vi "CSM - Data Type.vi"(8 "error in (no error)":errorcluster, 11 "variant":variant) -> (0 "error out":errorcluster, 3 "Data Type String":string)   [LabVIEW 2017, in "CSM MassData Parameter Support.lvlib"]
uses:
  CSM MassData Parameter Support.lvlib
  <vilib>/Utility/Data Type/Type Definitions/Data Type.ctl
  <vilib>/Utility/Data Type/NI_Data Type.lvlib
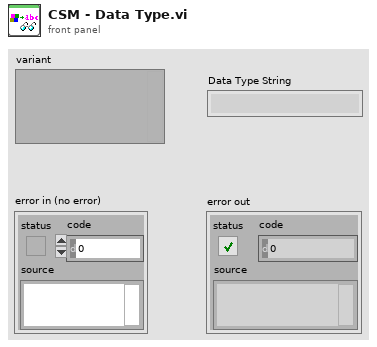
[diagram p1: front panel]
types:
  T1 = typedef "NI_Data Type.lvlib/Data Type.ctl" = enum8{"Invalid Type", "Void", "I8", "I16", "I32", "I64", "U8", "U16", "U32", "U64", "Single Float", "Double Float", "Extended Float", "Single Complex", "Double Complex", "Extended Complex", "Enum U8", "Enum U16", "Enum U32", "Enum U64", "Single Float With Unit", "Double Float With Unit", "Extended Float With Unit", "Single Complex with Unit", "Double Complex with Unit", "Extended Complex with Unit", "Boolean", "String", "Path", "Picture", "Tag", "Array", "Cluster", "Variant", "LV Variant", "Waveform", "Timestamp", "Digital Waveform", "Digital Data", "ExpressData", "Refnum", "External Data", "VI", "Poly VI", "LabVIEW Class Instance", "Fixed Point"}
  T2 = typedef "NI_Data Type.lvlib/Refnum Type.ctl" = enum16{"NotARefnum", "UnknownRefnum", "Generic", "Datalog", "ByteStream", "Device", "Occurence", "TCPNetConnection", "Auto", "Menu", "Imaq", "Hardware", "DataSocket", "Visa", "IVI", "UDPNetConnection", "Notifier", "Queue", "Irda", "EventReg", "DotNet", "UserEvent", "Callback", "UNUSED_EMPTY_POSITION", "BlueToothNetConnection", "LVObjApp", "LVObjVI", "LVObjUnknown", "GenericClass", "UserDefinedRefnumTag", "DataValue", "RT FIFO", "TDMS File"}
  T3 = typedef "NI_Data Type.lvlib/Tag Type.ctl" = enum16{"kNoTagType", "\tkDSCTagType", "\tkOldDAQTagType", "\tkIVITagType", "\tkVISATagType", "\tkGenClassTagType", "\tkUnusedTagType1", "\tkFPTagType", "\tkMotionTagType", "\tkDAQmxTaskTagType", "\tkDAQmxChannelTagType", "\tkDAQmxScaleTagType", "\tkDAQmxDeviceTagType", "\tkDAQmxTerminalTagType", "\tkDAQmxPhysChanTagType", "\tkDAQmxTriggerTagType", "\tkDAQmxSwitchTagType", "\tkDAQmxSignalTagType", "\tkUnusedTagType2", "\tkCANTaskTagType", "\tkCANInterfaceTagType", "\tkCANChannelTagType", "\tkNumTagTypes"}
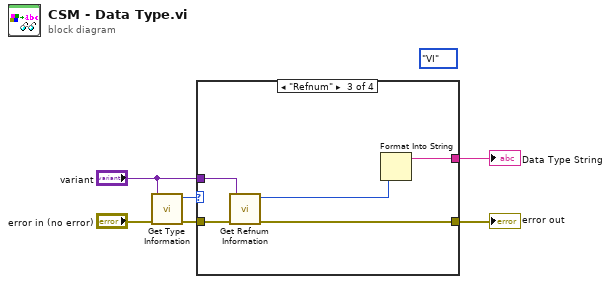
[diagram p0: block diagram]
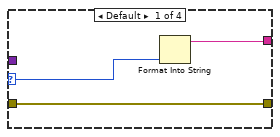
[diagram p2: hidden frame]
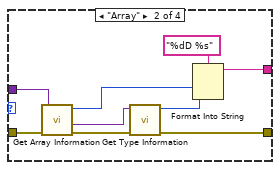
[diagram p3: hidden frame]
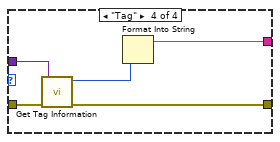
[diagram p4: hidden frame]
diagram:
  (unwired) Data_Type."VI" ("type")
  n1 = call <vilib>:"Get Type Information.vi"("error in (no error)"="error in (no error)", "Variant"="variant") -> ("error out"=w5:errorcluster, "Type"=w6:T1)  [unwired: 5 in, 3 out]
  n2 = case shown="\"Refnum\"" w6 {
    selector: w6 -> [w8 _ _ _]
    tunnel: w5 -> [w7 w18 w23 w28]
    tunnel: "variant" -> [_ w17 w22 w27]
    tunnel: [w9 w11 w19 w24] -> w3
    tunnel: [w7 w10 w21 w26] -> w1
    frame Default {
      n3 = Format Into String(w8) -> (resulting string=w9:string)  [unwired: 3 in, 1 out]
    }
    frame "Array" {
      n4 = call <vilib>:"Get Array Information.vi"("error in (no error)"=w18, "Variant"=w17) -> ("error out"=w16:errorcluster, "Array Element Data Type"=w13:variant, "Number of Dimensions"=w15:i32)  [unwired: 6 in, 1 out]
      n5 = call <vilib>:"Get Type Information.vi"("error in (no error)"=w16, "Variant"=w13) -> ("error out"=w10:errorcluster, "Type"=w12:T1)  [unwired: 5 in, 3 out]
      n6 = Format Into String(format string="%dD %s", w15, w12) -> (resulting string=w11:string)  [unwired: 2 in, 1 out]
    }
    frame "Refnum" {
      n7 = call <vilib>:"Get Refnum Information.vi"("error in (no error)"=w23, "Variant"=w22) -> ("error out"=w21:errorcluster, "Reference Type"=w20:T2)  [unwired: 6 in, 2 out]
      n8 = Format Into String(w20) -> (resulting string=w19:string)  [unwired: 3 in, 1 out]
    }
    frame "Tag" {
      n9 = call <vilib>:"Get Tag Information.vi"("error in (no error)"=w28, "Variant"=w27) -> ("error out"=w26:errorcluster, "Tag Type"=w25:T3)  [unwired: 8 in]
      n10 = Format Into String(w25) -> (resulting string=w24:string)  [unwired: 3 in, 1 out]
    }
  }
  "Data Type String" <- w3
  "error out" <- w1
